vi "Get Relay numbers 327-LEPL-104-M.vi"(8 "error in (no error)":errorcluster) -> (0 "error out":errorcluster, 2 "DUT2":T1, 3 "DUT1":T1)   [LabVIEW 2023]
uses:
  DUT_Relays_327-LEPL-104-M.ctl
  <vilib>/Utility/config.llb/Read Key (U32).vi
  <vilib>/Utility/config.llb/NI_LVConfig.lvlib
panel:
  out "error IO":errorcluster
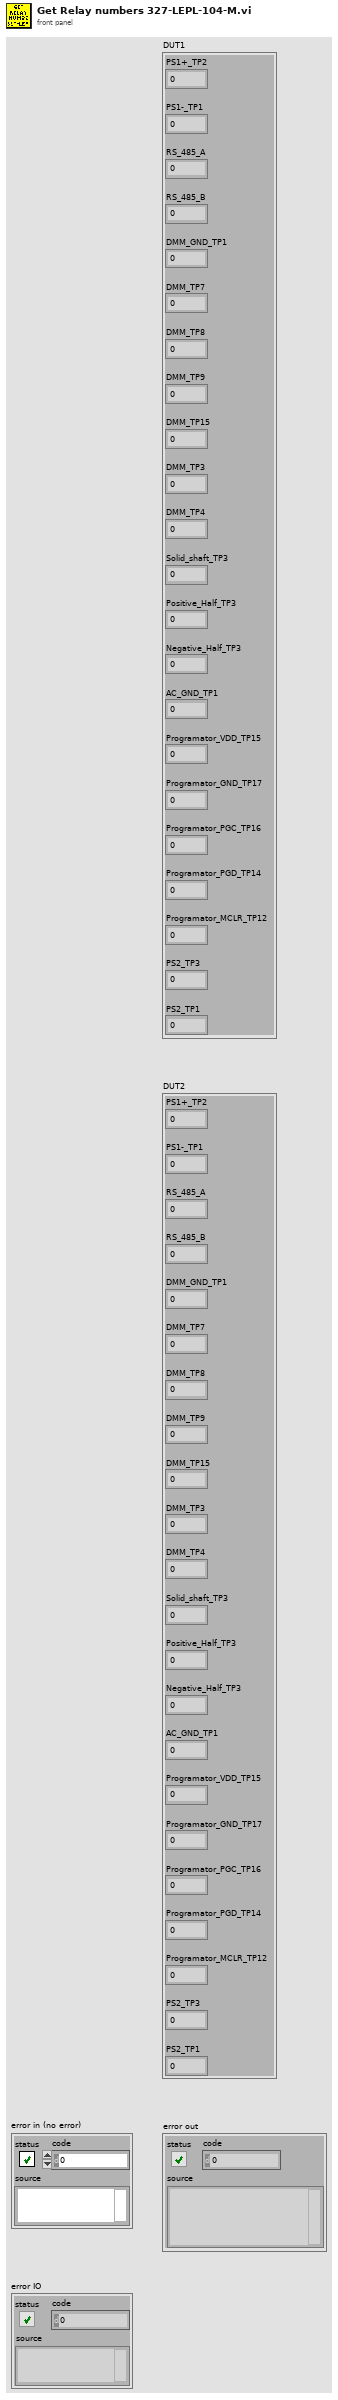
[diagram p1: front panel]
types:
  T1 = typedef "DUT_Relays_327-LEPL-104-M.ctl" = cluster{"PS1+_TP2":i32, "PS1-_TP1":i32, "RS_485_A":i32, "RS_485_B":i32, "DMM_GND_TP1":i32, "DMM_TP7":i32, "DMM_TP8":i32, "DMM_TP9":i32, "DMM_TP15":i32, "DMM_TP3":i32, "DMM_TP4":i32, "Positive_Half_TP3":i32, "Negative_Half_TP3":i32, "Solid_shaft_TP3":i32, "AC_GND_TP1":i32, "Programator_VDD_TP15 ":i32, "Programator_GND_TP17":i32, "Programator_PGC_TP16":i32, "Programator_PGD_TP14":i32, "Programator_MCLR_TP12":i32, "PS2_TP3":i32, "PS2_TP1":i32}
  T2 = typedef "NI_LVConfig.lvlib/Config Data RefNum.ctl" = refnum<k1>
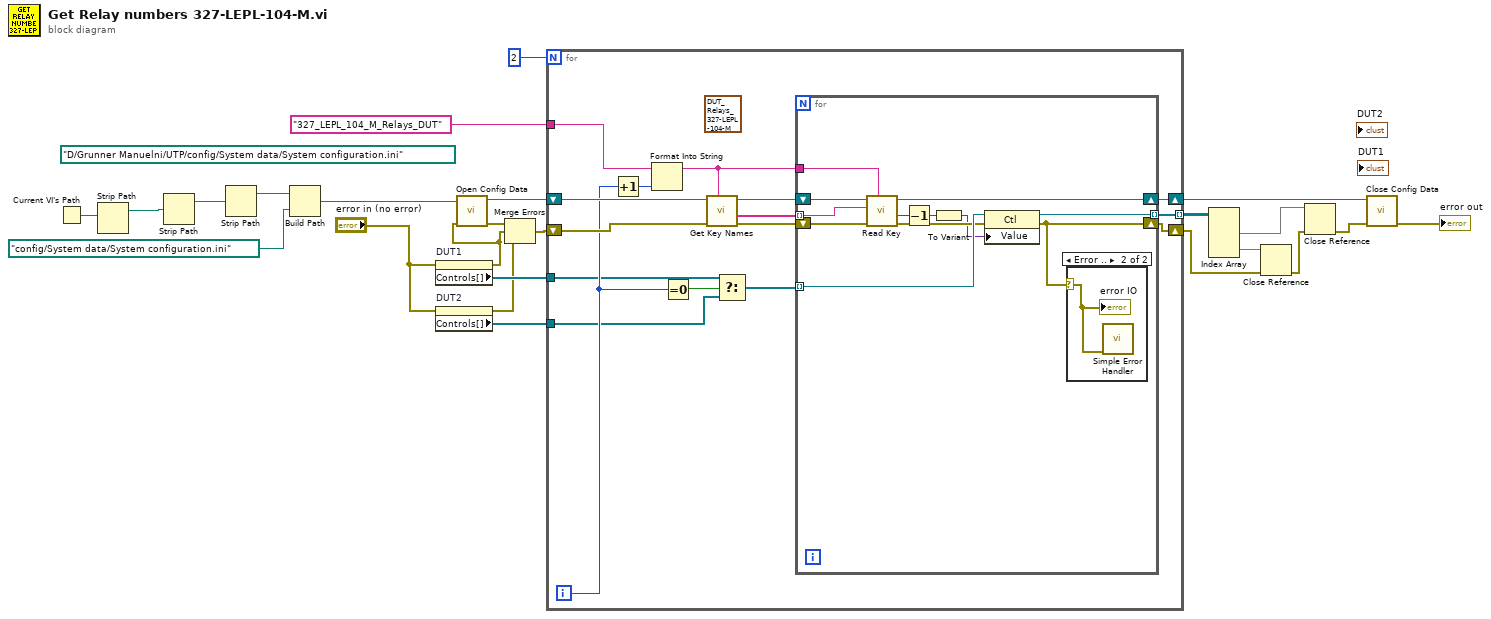
[diagram p0: block diagram]
diagram:
  (unwired) path "D:/Grunner Manuelni/UTP/config/System data/System configuration.ini" ("configuration file path")
  n1 = Current VI's Path() -> (path=w5:path)
  n2 = Strip Path(path=w5) -> (stripped path=w4:path)  [unwired: 1 out]
  n3 = Strip Path(path=w4) -> (stripped path=w8:path)  [unwired: 1 out]
  n4 = Strip Path(path=w8) -> (stripped path=w7:path)  [unwired: 1 out]
  n5 = Build Path(base path=w7, name or relative path=path "config/System data/System configuration.ini") -> (appended path=w3:path)
  n6 = property on="DUT1" class="Clust (strict)"(error in="error in (no error)") -> (error out=w1:errorcluster, "Controls[]"=w19:refnum<vi>[])  [unwired: 1 in, 1 out]
  n7 = property on="DUT2" class="Clust (strict)"(error in="error in (no error)") -> (error out=w15:errorcluster, "Controls[]"=w18:refnum<vi>[])  [unwired: 1 in, 1 out]
  n8 = call <vilib>:"Open Config Data.vi"("error in (no error)"=w1, "configuration file path"=w3) -> ("error out"=w16:errorcluster, "refnum"=w24:T2)  [unwired: 7 in, 1 out]
  n9 = Merge Errors(w16, w1, w15) -> (w17:errorcluster)
  n10 = for {
    N: 2 -> [_]
    shift-right: [w34] -> w23
    shift-left: w24 -> [w40]
    shift-right: [w35] -> w9
    shift-left: w17 -> [w37]
    tunnel: w19 -> [w30]
    tunnel: w18 -> [w27]
    tunnel: [w26] -> w13 mode=indexing
    tunnel: "327_LEPL_104_M_Relays_DUT" ("section") -> [w25]
    i -> [w31]
    (unwired) T1 {"PS1+_TP2"=0, "PS1-_TP1"=0, "RS_485_A"=0, "RS_485_B"=0, "DMM_GND_TP1"=0, "DMM_TP7"=0, "DMM_TP8"=0, "DMM_TP9"=0, "DMM_TP15"=0, "DMM_TP3"=0, "DMM_TP4"=0, "Positive_Half_TP3"=0, "Negative_Half_TP3"=0, "Solid_shaft_TP3"=0, "AC_GND_TP1"=0, "Programator_VDD_TP15 "=0, "Programator_GND_TP17"=0, "Programator_PGC_TP16"=0, "Programator_PGD_TP14"=0, "Programator_MCLR_TP12"=0, "PS2_TP3"=0, "PS2_TP1"=0} ("DUT1")
    n11 = Increment(x=w31) -> (x+1=w33:i32)
    n12 = Format Into String(initial string=w25, w33) -> (resulting string=w32:string)  [unwired: 2 in, 1 out]
    n13 = Equal To 0?(x=w31) -> (x = 0?=w28:bool)
    n14 = call <vilib>:"Get Key Names.vi"("section"=w32, "error in (no error)"=w37, "refnum"=w40) -> ("error out"=w36:errorcluster, "key names"=w39:string[], "refnum out"=w38:T2)  [unwired: 5 in, 1 out]
    n15 = Select(t=w30, s=w28, f=w27) -> (s? t:f=w29:refnum<vi>[])
    n16 = for {
      tunnel: w39 -> [w50] mode=indexing
      shift-right: [w51] -> w34
      shift-left: w38 -> [w52]
      tunnel: w32 -> [w49]
      tunnel: w29 -> [w47] mode=indexing
      tunnel: [w43] -> w26 mode=indexing
      shift-right: [w42] -> w35
      shift-left: w36 -> [w48]
      n17 = call-poly <vilib>:"Read Key.vi"("section"=w49, "error in (no error)"=w48, "key"=w50, "refnum"=w52) -> ("error out"=w46:errorcluster, "value"=w45:u32, "refnum out"=w51:T2)  [unwired: 4 in, 1 out]
      n18 = Decrement(x=w45) -> (x-1=w41:u32)
      n19 = To Variant(anything=w41) -> (Variant=w44:variant)
      n20 = property class="Ctl"(reference=w47, error in=w46, "Value"=w44) -> (reference out=w43:refnum<vi>, error out=w42:errorcluster)
      n21 = case shown="Error .." w42 {
        selector: w42 -> [_ w53]
        frame No Error {
        }
        frame Error {
          n22 = call <vilib>:"Simple Error Handler.vi"("error in (no error)"=w53) -> ()  [unwired: 4 in, 5 out]
          "error IO" <- w53
        }
      }
    }
  }
  n23 = Index Array(array=w13) -> (element #1=w12:refnum<vi>[], element #2=w11:refnum<vi>[])  [unwired: 4 in]
  n24 = Close Reference(reference=w11, error in (no error)=w9) -> (error out=w10:errorcluster)
  n25 = Close Reference(reference=w12, error in (no error)=w10) -> (error out=w22:errorcluster)
  n26 = call <vilib>:"Close Config Data.vi"("error in (no error)"=w22, "refnum"=w23) -> ("error out"=→"error out":errorcluster)  [unwired: 8 in, 1 out]
